vi "Simulation Lab -quad eqn - B220061.vi"() -> ()   [LabVIEW 2020]
panel:
  out "y":dbl
  in  "x":dbl
  in  "c":dbl
  in  "b":dbl
  in  "a":dbl
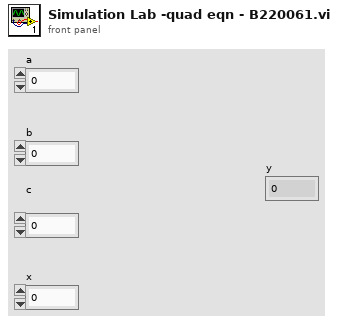
[diagram p1: front panel]
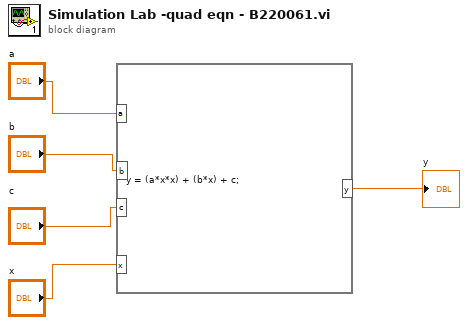
[diagram p0: block diagram]
diagram:
  n1 = formula code="y = (a*x*x) + (b*x) + c;"("a"="a", "x"="x", "b"="b", "c"="c") -> ("y"=→"y":dbl)
